vi "qSCT.vi"(0 "System no.":i32=1 min=1 max=4 step=1, 5 "error in":errorcluster) -> (14 "Cycle time, ms":i32, 19 "error out":errorcluster)   [LabVIEW 2020]
doc: "Returns current cycle time for MOV! command.\n\nC-887, F-206, M-8X0: For GCS syntax version = GCS 1.0 (Check with CSV?.vi. If CSV?.vi is not supported, syntax version is GCS 1.0), returns cycle time for MOV! command.\nFor GCS 2.0 or higher, returns cycle time for MOV command. Parameter 0x19001900 must be set to 1 in this case (SPA.vi), see controller user manual for details."
panel:
  # "Returns current cycle time for MOV! command in msec."
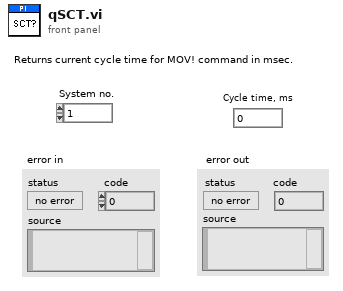
[diagram p1: front panel]
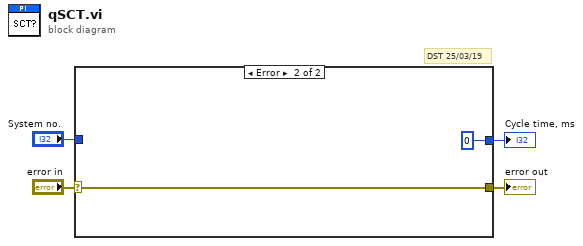
[diagram p0: block diagram]
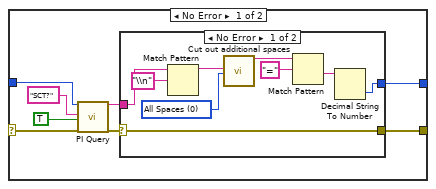
[diagram p2: hidden frame]
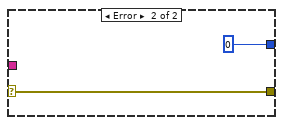
[diagram p3: hidden frame]
diagram:
  # "DST 25/03/19"
  n1 = case shown="Error" "error in" {
    selector: "error in" -> [w7 w24]
    tunnel: [w12 0] -> w4
    tunnel: "System no." -> [w10 _]
    tunnel: [w5 w24] -> w2
    frame No Error {
      n2 = call "PI Query.vi"("System no."=w10, "String to send"="SCT?", "Attach termination char.?"=TRUE ("Attach Linefeed?"), "error in"=w7) -> ("String read"=w8:string, "error out"=w6:errorcluster)  [unwired: 3 in, 11 out]
      n3 = case shown="No Error" w6 {
        selector: w6 -> [w13 w22]
        tunnel: w8 -> [w20 _]
        tunnel: [w21 0] -> w12
        tunnel: [w13 w22] -> w5
        frame No Error {
          w17 = u16 0 items=["All Spaces", "Only if 1st char.", "Only if last char.", "Only if near \"=\"", "Only if 1st or last char.", "Only multiple", "Really all"] ("Mode")
          n4 = Match Pattern(string=w20, regular expression="\\n") -> (before substring=w18:string)  [unwired: 4 out]
          n5 = call "Cut out additional spaces.vi"("String"=w18, "Mode"=w17) -> ("String out"=w16:string)  [unwired: 17 out]
          n6 = Match Pattern(string=w16, regular expression="=") -> (after substring=w14:string)  [unwired: 4 out]
          n7 = Decimal String To Number(string=w14) -> (number=w21:i32)  [unwired: 3 out]
        }
        frame Error {
        }
      }
    }
    frame Error {
    }
  }
  "error out" <- w2
  "Cycle time, ms" <- w4
